vi "Set Variables.vi"(8 "error in (no error)":errorcluster, 11 "Data":T1) -> (0 "error out":errorcluster)   [LabVIEW 2025, in "Runtime Configuration Support Example Engine.lvlib"]
uses:
  Runtime Configuration Support Example Engine.lvlib
  HW Operations.ctl
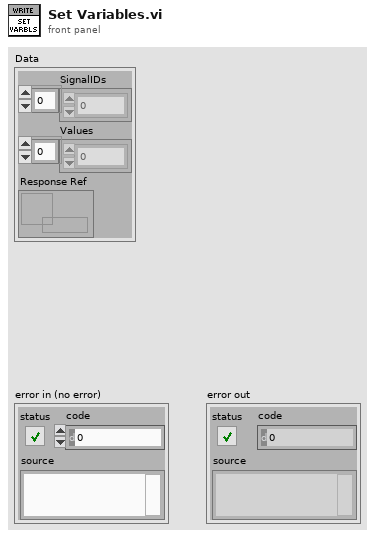
[diagram p1: front panel]
types:
  T1 = cluster{"SignalIDs":i32[], "Values":i32[], "Response Ref":refnum<queue>}
  T2 = typedef "HW Operations.ctl" = enum16{"Initialize", "Set In Val", "Get In Val", "Set Block", "Set Out Val", "Get Out Val", "Get In Array", "Get Out Array"}
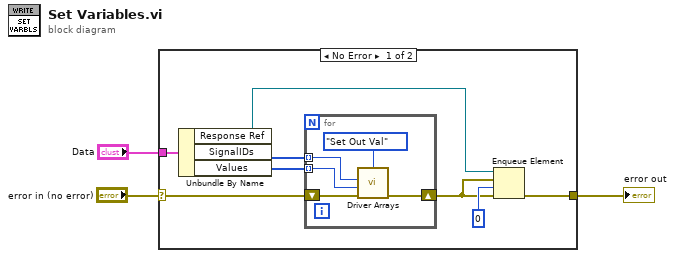
[diagram p0: block diagram]
diagram:
  n1 = case shown="No Error" "error in (no error)" {
    selector: "error in (no error)" -> [w5 w17]
    tunnel: [w4 w17] -> w3
    tunnel: "Data" -> [w11 _]
    frame No Error {
      n2 = Unbundle By Name(w11) -> ("Response Ref"=w9:refnum<queue>, "SignalIDs"=w10:i32[], "Values"=w8:i32[])
      n3 = for {
        tunnel: w10 -> [w13] mode=indexing
        shift-right: [w15] -> w6
        shift-left: w5 -> [w16]
        tunnel: w8 -> [w12] mode=indexing
        n4 = call "Driver Arrays.vi"("error in"=w16, "Value"=w12, "Index"=w13, "Curr Operation"=HW_Operations."Set Out Val") -> ("error out"=w15:errorcluster)  [unwired: 4 in, 3 out]
      }
      n5 = Enqueue Element(queue=w9, element=w6, timeout in ms (-1)=0, error in (no error)=w6) -> (error out=w4:errorcluster)  [unwired: 2 out]
    }
    frame Error {
    }
  }
  "error out" <- w3
